vi "Set Title.vi"(8 "error in (no error)":errorcluster, 10 "Title":string="Override \"Set Title.vi\" to change", 11 "MainController in":refnum<class "MainController.lvclass">) -> (0 "error out":errorcluster, 3 "MainController out":refnum<class "MainController.lvclass">)   [LabVIEW 2012, in "Win8uiFramework.lvlib" / "MainController.lvclass"]
uses:
  MainController.lvclass
  MainController.lvclass/MainController.ctl
  ViewableActor.lvclass/ViewableActor.ctl
  Read Title Ref.vi
  Read UI VI Ref.vi
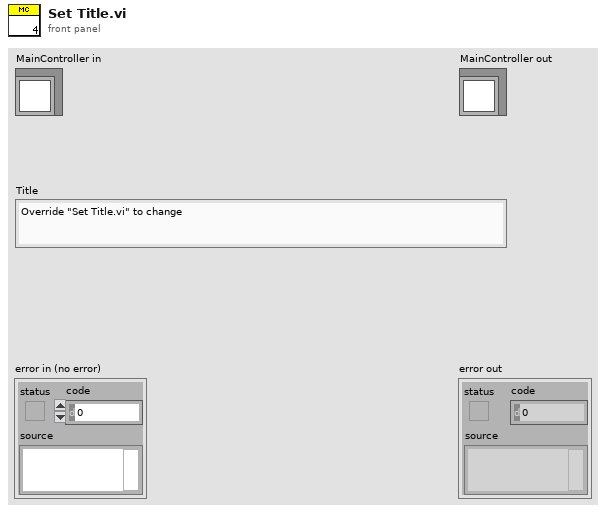
[diagram p1: front panel]
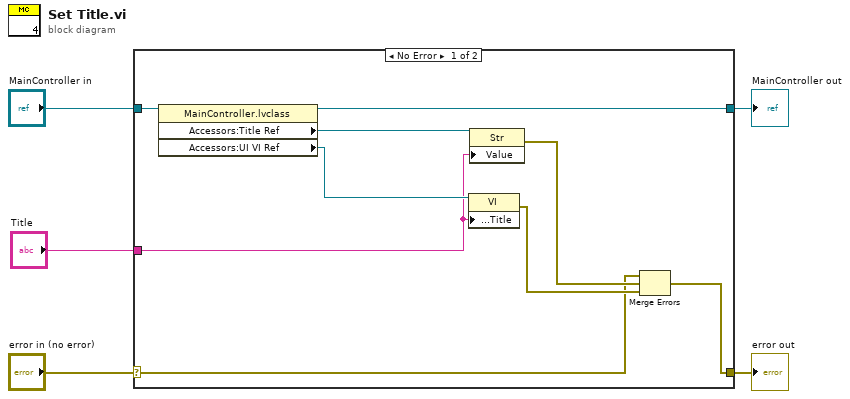
[diagram p0: block diagram]
diagram:
  n1 = case shown="No Error" "error in (no error)" {
    selector: "error in (no error)" -> [w8 w16]
    tunnel: [w7 w16] -> w4
    tunnel: [w13 w15] -> w2
    tunnel: "MainController in" -> [w14 w15]
    tunnel: "Title" -> [w6 _]
    frame No Error {
      n2 = property class="MainController.lvclass"(reference=w14) -> (reference out=w13:refnum<class "MainController.lvclass">, "Accessors:Title Ref"=w11:refnum<vi>, "Accessors:UI VI Ref"=w12:refnum<vi>)  [unwired: 1 in, 1 out]
      n3 = property class="VI"(reference=w12, "Front Panel.Title"=w6) -> (error out=w9:errorcluster)  [unwired: 1 in, 1 out]
      n4 = property class="Str"(reference=w11, "Value"=w6) -> (error out=w10:errorcluster)  [unwired: 1 in, 1 out]
      n5 = Merge Errors(w8, w10, w9) -> (w7:errorcluster)
    }
    frame Error {
    }
  }
  "error out" <- w4
  "MainController out" <- w2
